vi "do all three.vi"(6 "Gyro Target":dbl, 7 "Max Time":dbl, 8 "X Target":dbl, 9 "Y Target":dbl, 10 "Encoders In":T1, 11 "PID Gains In":T2={"X PID"={"proportional gain (Kc)"=0.02000000000000001, "integral time (Ti, min)"=0.0, "derivative time (Td, min)"=0.0}, "Y PID"={"proportional gain (Kc)"=0.02000000000000001, "integral time (Ti, min)"=0.0, "derivative time (Td, min)"=0.0}, "Z PID"={"proportional gain (Kc)"=0.02000000000000001, "integral time (Ti, min)"=0.0, "derivative time (Td, min)"=0.0}} {"Z PID"."derivative time (Td, min)" format="%.3f"; "Z PID"."integral time (Ti, min)" format="%.3f"; "Z PID"."proportional gain (Kc)" format="%.3f"; "Y PID"."derivative time (Td, min)" format="%.3f"; "Y PID"."integral time (Ti, min)" format="%.3f"; "Y PID"."proportional gain (Kc)" format="%.3f"; "X PID"."derivative time (Td, min)" format="%.3f"; "X PID"."integral time (Ti, min)" format="%.3f"; "X PID"."proportional gain (Kc)" format="%.3f"}) -> (2 "Encoders Out":T1, 3 "PID Gains Out":T2={"X PID"={"proportional gain (Kc)"=0.02000000000000001, "integral time (Ti, min)"=0.0, "derivative time (Td, min)"=0.0}, "Y PID"={"proportional gain (Kc)"=0.02000000000000001, "integral time (Ti, min)"=0.0, "derivative time (Td, min)"=0.0}, "Z PID"={"proportional gain (Kc)"=0.02000000000000001, "integral time (Ti, min)"=0.0, "derivative time (Td, min)"=0.0}} {"Z PID"."derivative time (Td, min)" format="%.3f"; "Z PID"."integral time (Ti, min)" format="%.3f"; "Z PID"."proportional gain (Kc)" format="%.3f"; "Y PID"."derivative time (Td, min)" format="%.3f"; "Y PID"."integral time (Ti, min)" format="%.3f"; "Y PID"."proportional gain (Kc)" format="%.3f"; "X PID"."derivative time (Td, min)" format="%.3f"; "X PID"."integral time (Ti, min)" format="%.3f"; "X PID"."proportional gain (Kc)" format="%.3f"})   [LabVIEW 2018]
uses:
  <vilib>/addons/control/pid/pid.llb/PID (DBL).vi
  2019 Swerve Test Chassis/SwerveChassis2019Test 2.3/Robot Global Data.vi
  2.2/SubSystems/Robot Information/Robot Information Global.vi
  <vilib>/addons/control/pid/NI_PID_pid.lvlib
panel:
  in  "Movement":enum16{"0", "1", "2", "3", "4", "5"}(ring)
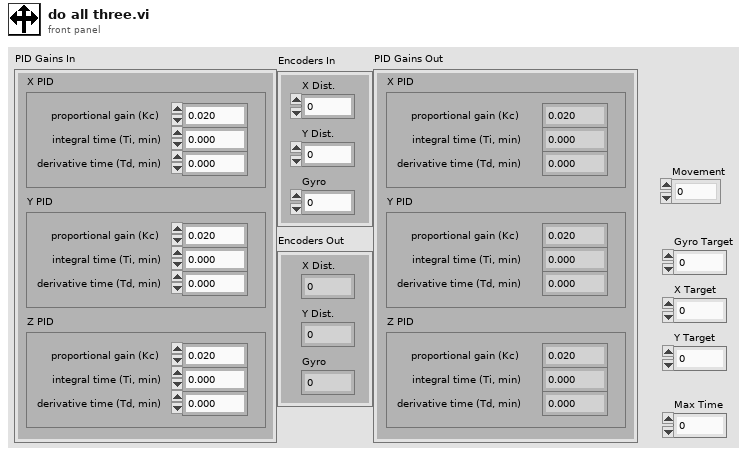
[diagram p1: front panel]
types:
  T1 = cluster{"X Dist.":dbl, "Y Dist.":dbl, "Gyro":dbl}
  T2 = cluster{"X PID":cluster{"proportional gain (Kc)":dbl, "integral time (Ti, min)":dbl, "derivative time (Td, min)":dbl}, "Y PID":cluster{"proportional gain (Kc)":dbl, "integral time (Ti, min)":dbl, "derivative time (Td, min)":dbl}, "Z PID":cluster{"proportional gain (Kc)":dbl, "integral time (Ti, min)":dbl, "derivative time (Td, min)":dbl}}
  T3 = cluster{"proportional gain (Kc)":dbl, "integral time (Ti, min)":dbl, "derivative time (Td, min)":dbl}
  T4 = enum16{"0", "1", "2", "3", "4", "5", "6", "7", "8", "9", "10", "11", "12", "13", "14", "15", "16"}
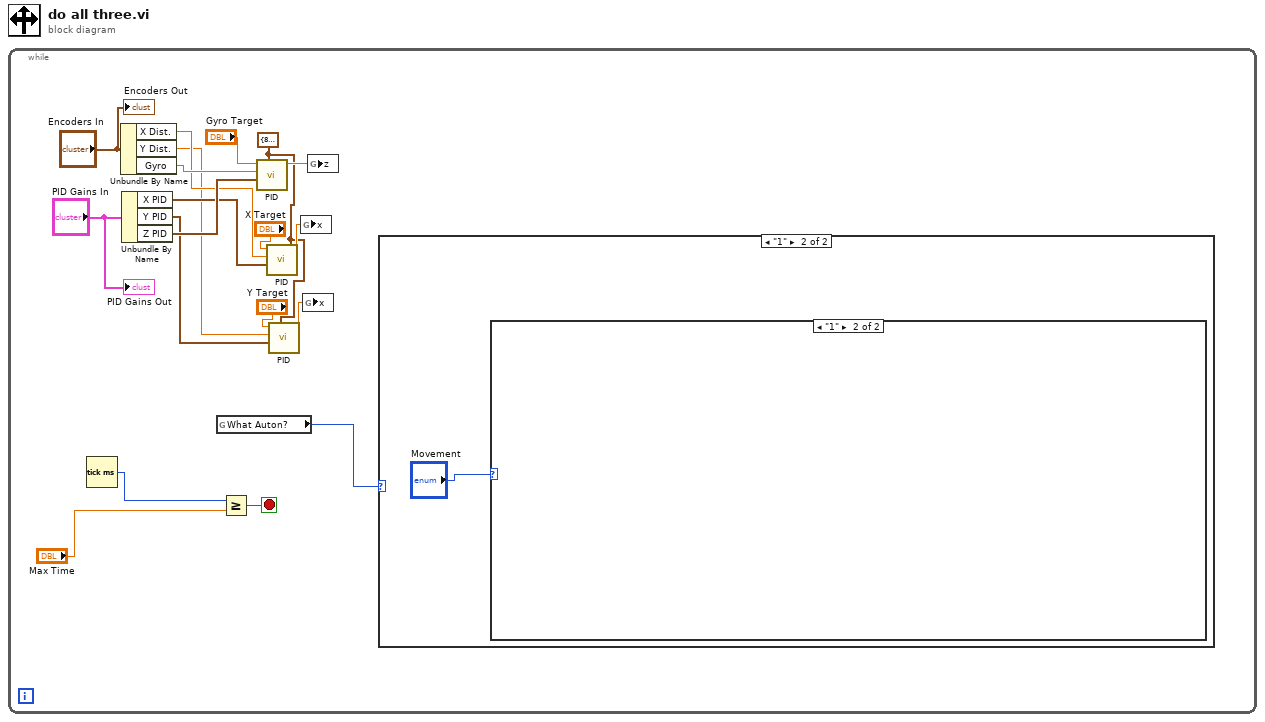
[diagram p0: block diagram]
diagram:
  n1 = while {
    stop <- w4 stop-if-true
    w5 = cluster{"output high":dbl, "output low":dbl} {"output high"=8.0, "output low"=-8.0} ("output range")
    n2 = Tick Count (ms)() -> (millisecond timer value=w3:u32)
    n3 = Unbundle By Name("Encoders In") -> ("X Dist."=w11:dbl, "Y Dist."=w6:dbl, "Gyro"=w15:dbl)
    n4 = Unbundle By Name("PID Gains In") -> ("X PID"=w13:T3, "Y PID"=w7:T3, "Z PID"=w14:T3)
    n5 = global read "Robot Information Global.vi" "What Auton?"() -> (w1:T4)
    n6 = Greater Or Equal?(x=w3, y="Max Time") -> (x >= y?=w4:bool)
    n7 = call-poly <vilib>:"PID.vi"("output range"=w5, "PID gains"=w14, "process variable"=w15, "setpoint"="Gyro Target") -> ("output"=w18:dbl)  [unwired: 6 in, 1 out]
    n8 = call-poly <vilib>:"PID.vi"("output range"=w5, "PID gains"=w13, "process variable"=w11, "setpoint"="X Target") -> ("output"=w12:dbl)  [unwired: 6 in, 1 out]
    n9 = call-poly <vilib>:"PID.vi"("output range"=w5, "PID gains"=w7, "process variable"=w6, "setpoint"="Y Target") -> ("output"=w8:dbl)  [unwired: 6 in, 1 out]
    n10 = global write "Robot Global Data.vi" "x"(w12) -> ()
    n11 = global write "Robot Global Data.vi" "x"(w8) -> ()
    n12 = global write "Robot Global Data.vi" "z"(w18) -> ()
    n13 = case shown="\"1\"" w1 {
      frame "0", Default {
      }
      frame "1" {
        n14 = case shown="\"1\"" "Movement" {
          frame "0", Default {
          }
          frame "1" {
          }
        }
      }
    }
    "PID Gains Out" <- "PID Gains In"
    "Encoders Out" <- "Encoders In"
  }
